vi "ParserEnum.vi"(8 "error in (no error)":errorcluster, 11 "JSON item":string) -> (0 "error out":errorcluster, 2 "enums":T1[](array[typedef]), 3 "JSON item":string)   [LabVIEW 2018, in "Paser.lvlib"]
uses:
  Paser.lvlib
  Ctrl/Enum.ctl
  Ctrl/EnumValue.ctl
  9c68dffb-d6a6-4821-96c9-585a19b7b73d.vi
  <vilib>/JDP Science/JSONtext/Find Item.vi
  <vilib>/JDP Science/JSONtext/String Subset.vi
  <vilib>/JDP Science/JSONtext/Parsing/Parse Full Path or Item Name.vi
  <vilib>/JDP Science/JSONtext/Offset/Find Item Locations by Path.vi
  <vilib>/JDP Science/JSONtext/JSON text to Variant.vi
  <vilib>/JDP Science/JSONtext/JSONtext.lvlib
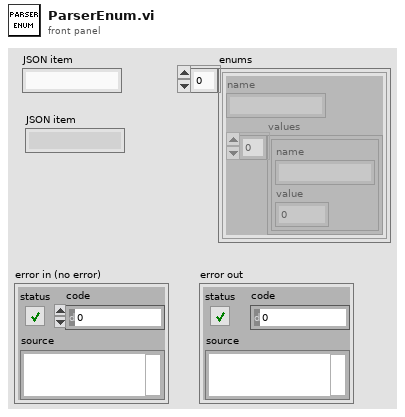
[diagram p1: front panel]
types:
  T1 = typedef "Enum.ctl" = cluster{"name":string, "values":T2[]}
  T2 = typedef "EnumValue.ctl" = cluster{"name":string, "value":i32}
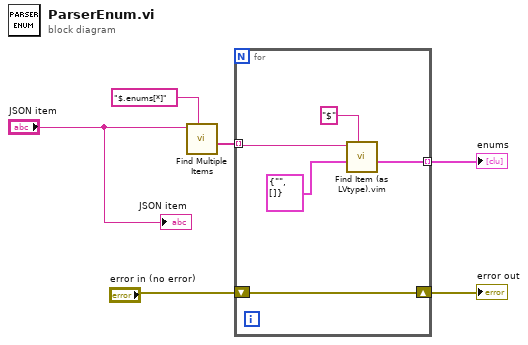
[diagram p0: block diagram]
diagram:
  n1 = call <vilib>:"Find Multiple Items.vi"("$Path or Item Name"="$.enums[*]", "JSON"="JSON item") -> ("<JSON>"=w4:string[])  [unwired: 6 in, 3 out]
  n2 = for {
    tunnel: w4 -> [w9] mode=indexing
    shift-right: [w7] -> w6
    shift-left: "error in (no error)" -> [w7]
    tunnel: [w8] -> w1 mode=indexing
    n3 = call "Find Item (as LVtype).vim"("$Path or Item Name"="$", "Data Type and Default Value"=T1 {"name"="", "values"=[]} ("Enum"), "JSON"=w9) -> ("Data"=w8:T1)  [unwired: 5 in, 3 out]
  }
  "error out" <- w6
  "enums" <- w1
  "JSON item" <- "JSON item"
